vi "Write Age.vi"(8 "error in (no error)":errorcluster, 10 "Age":i32, 11 "Atom in":refnum<class "Atom.lvclass">) -> (0 "error out":errorcluster, 3 "Atom out":refnum<class "Atom.lvclass">)   [LabVIEW 2020, in "Atom.lvclass"]
uses:
  Atom.lvclass
  Atom.lvclass/Atom.ctl
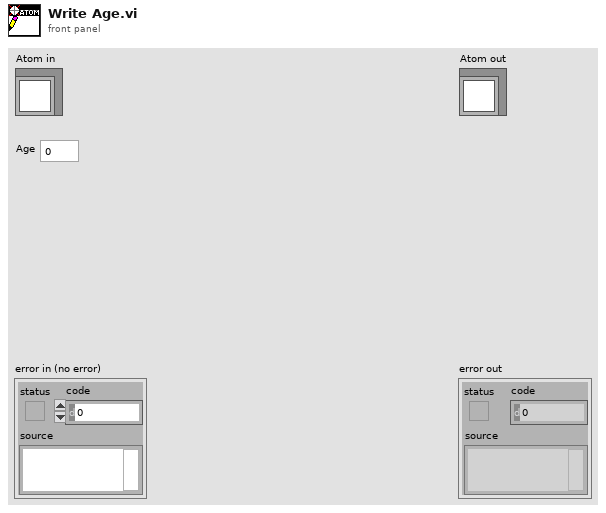
[diagram p1: front panel]
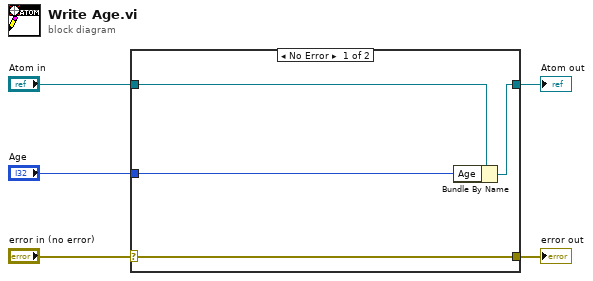
[diagram p0: block diagram]
diagram:
  n1 = case shown="No Error" "error in (no error)" {
    selector: "error in (no error)" -> [w9 w10]
    tunnel: [w9 w10] -> w4
    tunnel: [w7 w11] -> w2
    tunnel: "Atom in" -> [w8 w11]
    tunnel: "Age" -> [w6 _]
    frame No Error {
      n2 = Bundle By Name(cluster=w8, "Age"=w6) -> (w7:refnum<class "Atom.lvclass">)
    }
    frame Error {
    }
  }
  "error out" <- w4
  "Atom out" <- w2
